vi "Calibratore.vi"(8 "error in (no error)":errorcluster, 11 "VISA Refnum in":refnum<visa-resource-name>) -> (0 "error out":errorcluster, 2 "value":dbl, 3 "VISA Refnum out":refnum<visa-resource-name>)   [LabVIEW 2023]
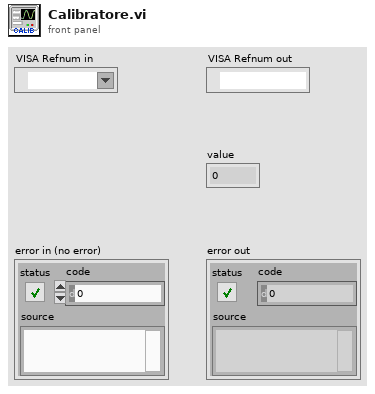
[diagram p1: front panel]
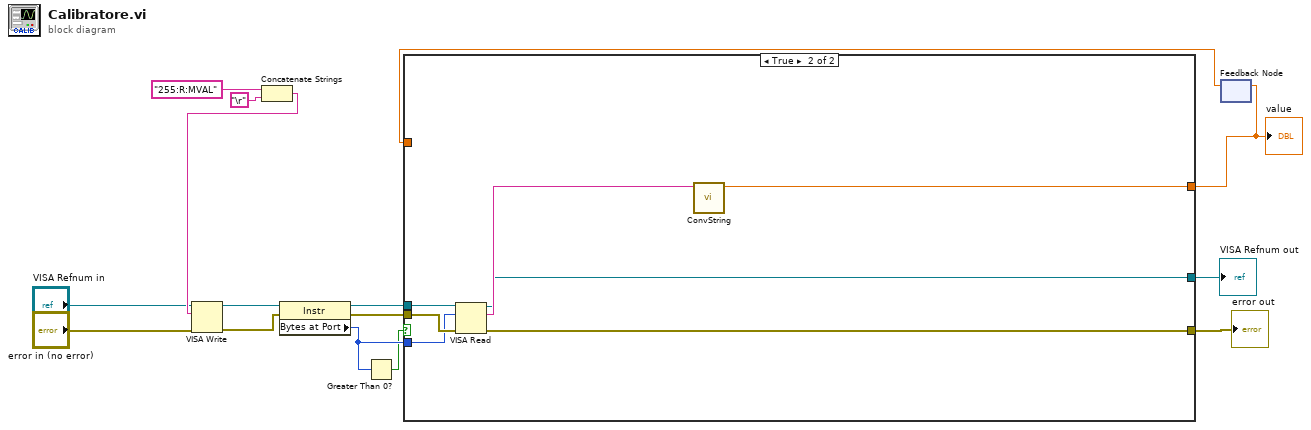
[diagram p0: block diagram]
diagram:
  n1 = Concatenate Strings("255:R:MVAL" ("write buffer"), "\r") -> (w15:string)
  n2 = VISA Write(VISA resource name="VISA Refnum in", write buffer=w15, error in (no error)="error in (no error)") -> (VISA resource name out=w4:refnum<visa-resource-name>, error out=w8:errorcluster)  [unwired: 1 out]
  n3 = property class="Instr"(reference=w4, error in=w8) -> (reference out=w6:refnum<visa-resource-name>, error out=w9:errorcluster, "Bytes at Port"=w12:u32)
  n4 = Greater Than 0?(x=w12) -> (x > 0?=w11:bool)
  n5 = feedback #1() -> (w1:dbl)  [unwired: 1 in]
  n6 = case shown="True" w11 {
    tunnel: w6 -> [w17 w25]
    tunnel: w9 -> [w18 w24]
    tunnel: [w18 w23] -> w10
    tunnel: w12 -> [_ w22]
    tunnel: [w16 w20] -> w2
    tunnel: [w17 w19] -> w3
    tunnel: w1 -> [w16 _]
    frame False {
    }
    frame True {
      n7 = VISA Read(VISA resource name=w25, byte count=w22, error in (no error)=w24) -> (VISA resource name out=w19:refnum<visa-resource-name>, read buffer=w21:string, error out=w23:errorcluster)  [unwired: 1 out]
      n8 = call "ConvString.vi"("read buffer"=w21) -> ("Numeric"=w20:dbl)  [unwired: 10 in]
    }
  }
  "error out" <- w10
  "value" <- w2
  "VISA Refnum out" <- w3
  n9 = feedback-in #1(w2) -> ()
